vi "Generate Random Gene.vi"(8 "error in":errorcluster, 11 "Real Gene in":refnum<class "Real Gene.lvclass">) -> (0 "error out":errorcluster, 3 "Real Gene out":refnum<class "Real Gene.lvclass">)   [LabVIEW 2016, in "Real Gene.lvclass"]
doc: "This VI generates a random Real-Valued Gene allele on the interval (0, 1] (Normal Distribution)\nThis is an overloaded VI of IGene method.\n\n**Author: Stas Legedza"
uses:
  Real Gene.lvclass
  Real Gene.lvclass/Real Gene.ctl
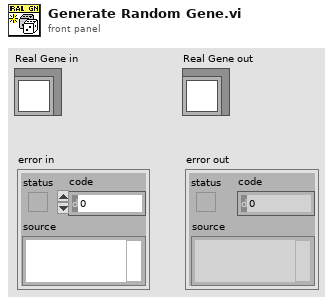
[diagram p1: front panel]
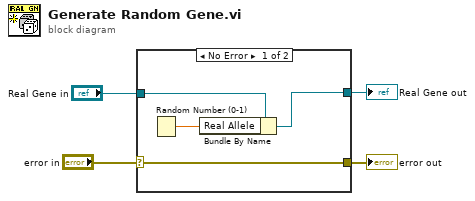
[diagram p0: block diagram]
diagram:
  n1 = case shown="No Error" "error in" {
    selector: "error in" -> [w5 w9]
    tunnel: "Real Gene in" -> [w8 w10]
    tunnel: [w7 w10] -> w2
    tunnel: [w5 w9] -> w1
    frame No Error {
      n2 = Random Number (0-1)() -> (number: 0 to 1=w6:dbl)
      n3 = Bundle By Name(cluster=w8, "Real Allele"=w6) -> (w7:refnum<class "Real Gene.lvclass">)
    }
    frame Error {
    }
  }
  "error out" <- w1
  "Real Gene out" <- w2
